vi "Game part 2.vi"() -> ()   [LabVIEW 2019]
uses:
  Control 1 State.ctl
  Control 2 App data.ctl
panel:
  in  "Type the sequence shown":T1
  out "Number of colours memorised 2":dbl
  in  "1":bool
  in  "0":bool
  in  "9":bool
  in  "6":bool
  in  "8":bool
  in  "7":bool
  in  "5":bool
  in  "4":bool
  in  "3":bool
  in  "2":bool
  out "Number of colours memorised":dbl
  out "Sequence to memorise":u32(colorbox)
  # "Memory Game"
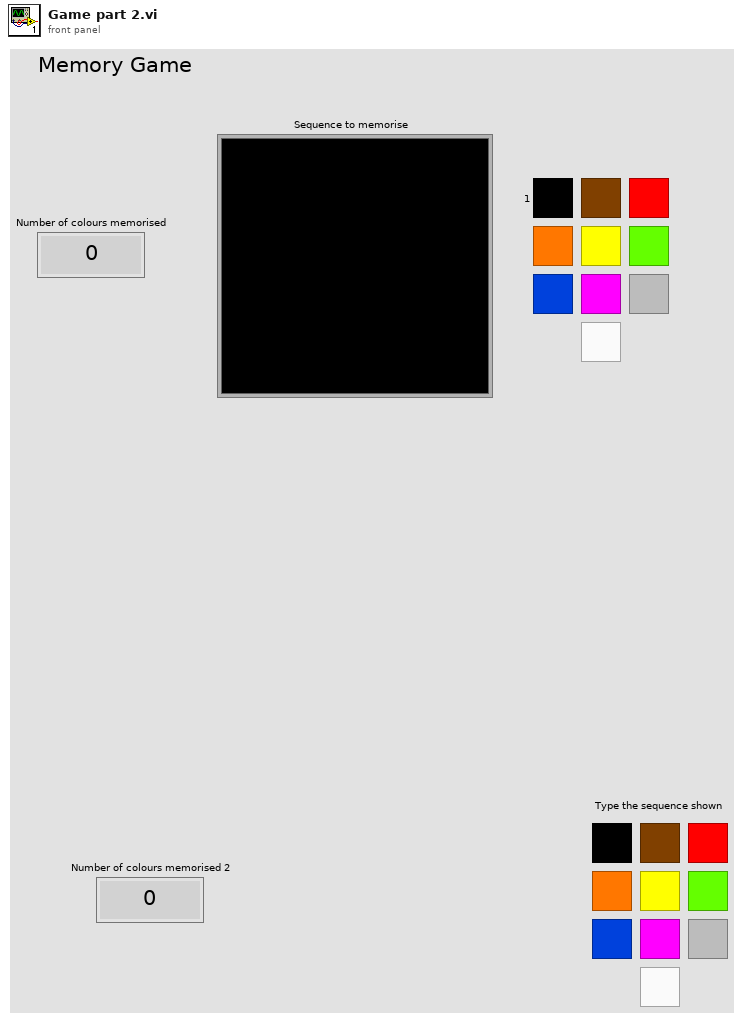
[diagram p1: front panel]
types:
  T1 = cluster{"0":bool, "1":bool, "2":bool, "3":bool, "4":bool, "5":bool, "6":bool, "7":bool, "8":bool, "9":bool}
  T2 = typedef "Control 2 App data.ctl" = cluster{"Sequence":i32[], "Colours":u32[], "Wait time (1*10^-3 s)":u32, "Last Key":i32, "No. Key presses":i32, "Tally":i32}
  T3 = typedef "Control 1 State.ctl" = enum16{"Initialize", "Add New Colour", "Show Sequence", "Wait For Event", "Check Key press", "Success", "Failure", "Exit"}
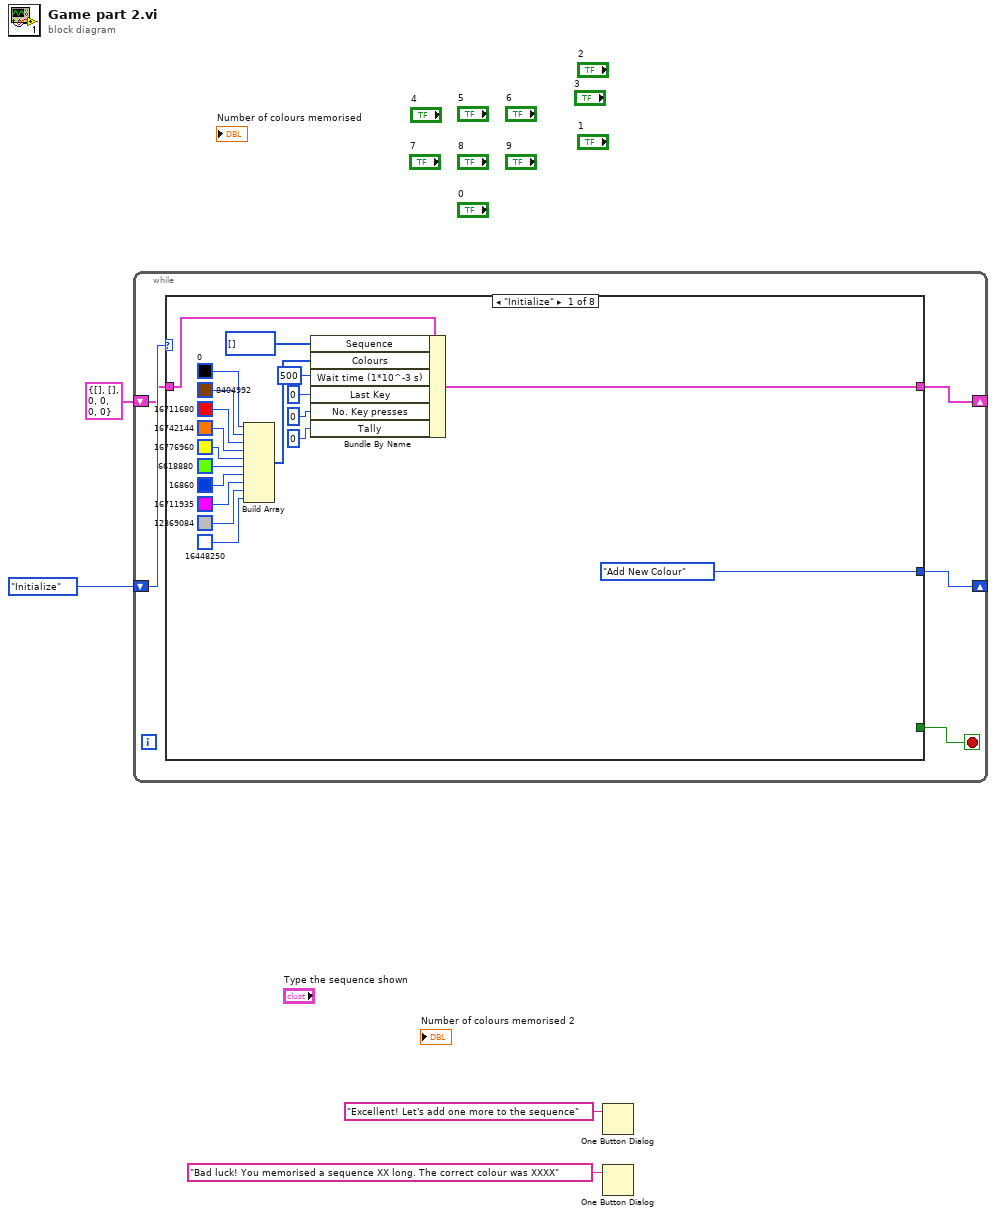
[diagram p0: block diagram]
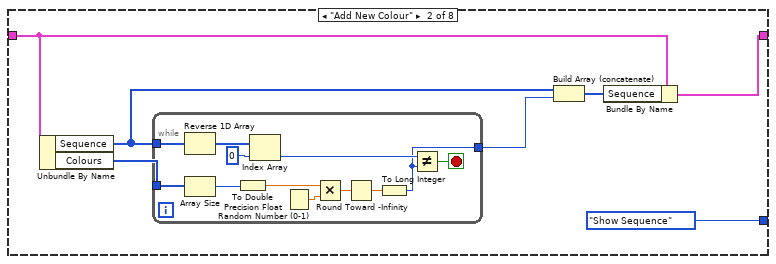
[diagram p2: hidden frame]
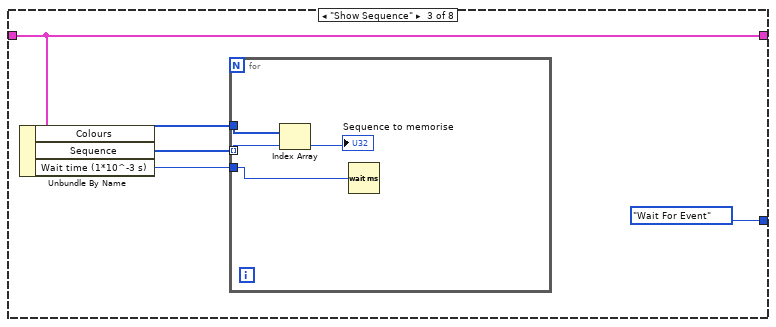
[diagram p3: hidden frame]
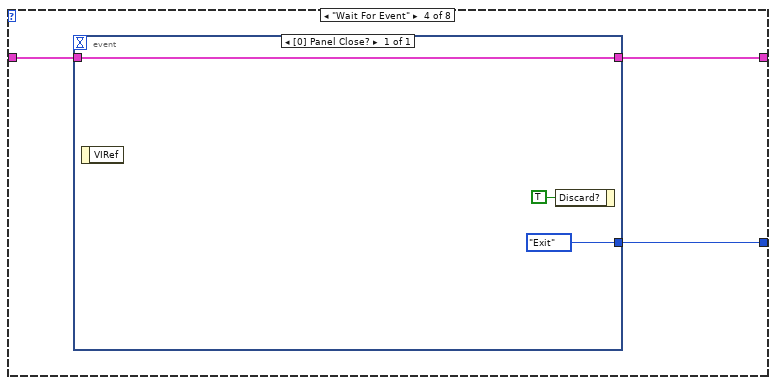
[diagram p4: hidden frame]
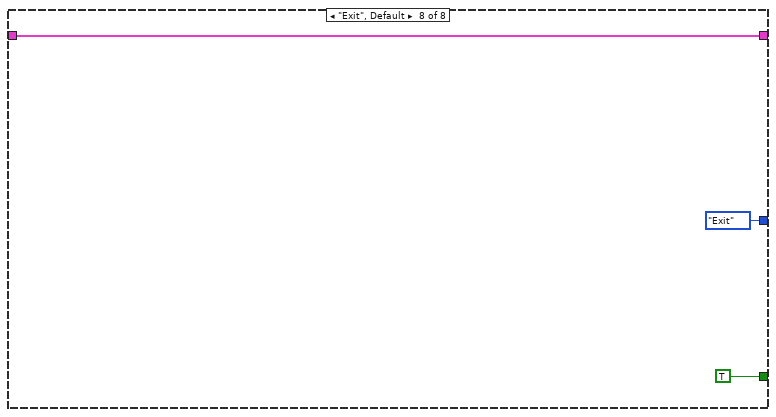
[diagram p8: hidden frame]
diagram:
  n1 = while {
    shift-right: [w7] -> _
    shift-left: T2 {"Sequence"=[], "Colours"=[], "Wait time (1*10^-3 s)"=0, "Last Key"=0, "No. Key presses"=0, "Tally"=0} -> [w8]
    shift-right: [w6] -> _
    shift-left: Control_1_State."Initialize" -> [w9]
    stop <- w5 stop-if-true
    n2 = case shown="\"Initialize\"" w9 {
      tunnel: w8 -> [w28 w31 w52 w59 w63 _ w64 w67]
      tunnel: [w27 w29 w52 _ w63 _ w64 w67] -> w7
      tunnel: [Control_1_State."Add New Colour" Control_1_State."Show Sequence" Control_1_State."Wait For Event" w57 _ _ _ Control_1_State."Exit"] -> w6
      tunnel: [_ _ _ w58 _ _ _ _] -> _
      tunnel: [_ _ _ _ _ _ _ TRUE] -> w5
      frame "Initialize" {
        n3 = Build Array(u32 0 ("Color Box"), u32 8404992 ("Color Box"), u32 16711680 ("Color Box"), u32 16742144 ("Color Box"), u32 16776960 ("Color Box"), u32 6618880 ("Color Box"), u32 16860 ("Color Box"), u32 16711935 ("Color Box"), u32 12369084 ("Color Box"), u32 16448250 ("Color Box")) -> (w12:u32[])
        n4 = Bundle By Name(cluster=w28, "Sequence"=i32[] [], "Colours"=w12, "Wait time (1*10^-3 s)"=u32 500, "Last Key"=0, "No. Key presses"=0, "Tally"=0) -> (w27:T2)
      }
      frame "Add New Colour" {
        n5 = Unbundle By Name(w31) -> ("Sequence"=w34:i32[], "Colours"=w35:u32[])
        n6 = while {
          tunnel: w34 -> [w47]
          tunnel: w35 -> [w44]
          tunnel: [w36] -> w33
          stop <- w37 stop-if-true
          n7 = Reverse 1D Array(array=w47) -> (reversed array=w46:i32[])
          n8 = Array Size(array=w44) -> (size(s)=w42:i32)
          n9 = To Double Precision Float(number=w42) -> (double precision float=w41:dbl)
          n10 = Index Array(array=w46, index=0) -> (element=w38:i32)
          n11 = Random Number (0-1)() -> (number: 0 to 1=w45:dbl)
          n12 = Multiply(x=w41, y=w45) -> (x*y=w43:dbl)
          n13 = Round Toward -Infinity(1:w43) -> (0:w39:dbl)
          n14 = To Long Integer(number=w39) -> (32bit integer=w36:i32)
          n15 = Not Equal?(x=w38, y=w36) -> (x != y?=w37:bool)
        }
        n16 = Build Array (concatenate)(w34, w33) -> (w32:i32[])
        n17 = Bundle By Name(cluster=w31, "Sequence"=w32) -> (w29:T2)
      }
      frame "Show Sequence" {
        n18 = Unbundle By Name(w52) -> ("Colours"=w50:u32[], "Sequence"=w51:i32[], "Wait time (1*10^-3 s)"=w49:u32)
        n19 = for {
          tunnel: w51 -> [w55] mode=indexing
          tunnel: w50 -> [w56]
          tunnel: w49 -> [w53]
          n20 = Index Array(array=w56, index=w55) -> (element=→"Sequence to memorise":u32)
          n21 = Wait (ms)(milliseconds to wait=w53) -> ()  [unwired: 1 out]
        }
      }
      frame "Wait For Event" {
        n22 = event shown="[0] Panel Close?" {
          selector: _ -> [_]
          dyn-events: _ -> [_]
          timeout: _ -> [_]
          tunnel: w59 -> [w62]
          tunnel: [w62] -> w58
          tunnel: [Control_1_State."Exit"] -> w57
          event Panel Close? {
            n23 = event-data() -> ()  [unwired: 1 in, 1 out]
            n24 = event-data("Discard?"=TRUE) -> ()  [unwired: 1 in, 1 out]
          }
        }
      }
      frame "Check Key press" {
      }
      frame "Success" {
      }
      frame "Failure" {
      }
      frame "Exit", Default {
      }
    }
  }
  n25 = One Button Dialog(message="Excellent! Let's add one more to the sequence") -> ()  [unwired: 1 in, 1 out]
  n26 = One Button Dialog(message="Bad luck! You memorised a sequence XX long. The correct colour was XXXX") -> ()  [unwired: 1 in, 1 out]
